vi "ConfirmReceipt.vi"(8 "error in (no error)":errorcluster, 9 "timeout in ms (10000)":i32=10000, 11 "STOMP in":refnum<class "STOMP.lvclass">) -> (0 "error out":errorcluster, 3 "STOMP out":refnum<class "STOMP.lvclass">)   [LabVIEW 2017, in "LabVIEW STOMP.lvlib" / "STOMP.lvclass"]
uses:
  STOMP.lvclass
  STOMP.lvclass/STOMP.ctl
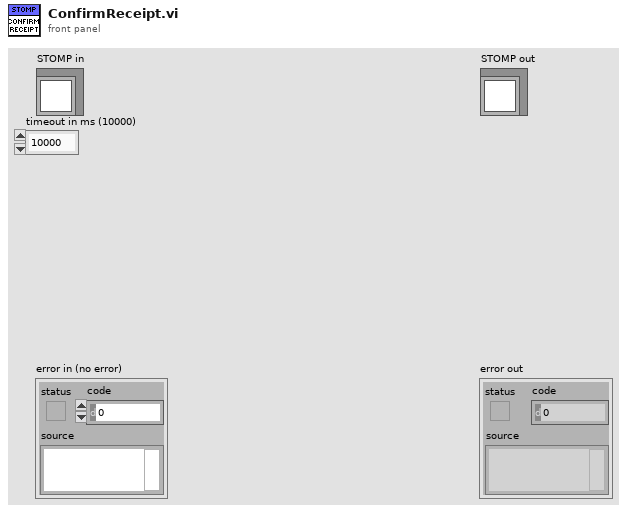
[diagram p1: front panel]
types:
  T1 = typedef "LabVIEW STOMP.lvlib/STOMP.lvclass/Type_ServerFrame.ctl" = cluster{"Type":T2, "Headers":cluster{"Header":string, "Value":string}[], "Body":string}
  T2 = typedef "LabVIEW STOMP.lvlib/STOMP.lvclass/Type_ServerFrameType.ctl" = enum16{"Undefined", "MESSAGE", "CONNECTED", "RECEIPT", "ERROR"}
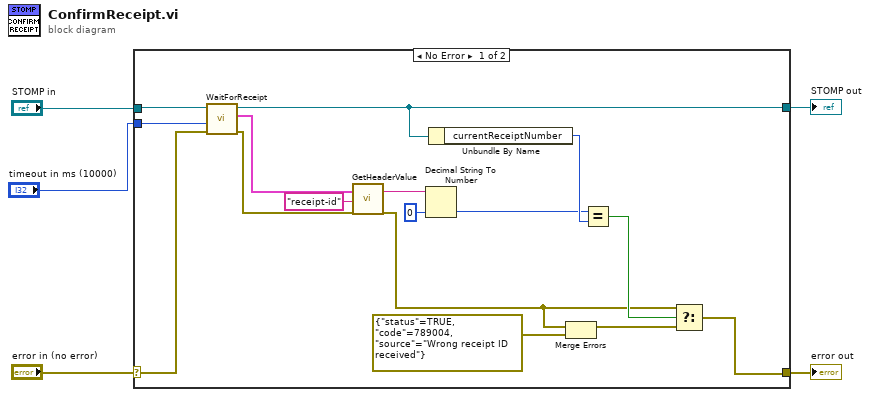
[diagram p0: block diagram]
diagram:
  n1 = case shown="No Error" "error in (no error)" {
    selector: "error in (no error)" -> [w20 w23]
    tunnel: [w6 w23] -> w4
    tunnel: [w14 w22] -> w2
    tunnel: "STOMP in" -> [w21 w22]
    tunnel: "timeout in ms (10000)" -> [w11 _]
    frame No Error {
      n2 = call-dynamic "WaitForReceipt.vi"("error in (no error)"=w20, "timeout in ms (10000)"=w11, "STOMP in"=w21) -> ("error out"=w18:errorcluster, "receipt"=w19:T1, "STOMP out"=w14:refnum<class "STOMP.lvclass">)  [unwired: 6 in]
      n3 = call "GetHeaderValue.vi"("Server Frame"=w19, "Header Name"="receipt-id", "error in"=w18) -> ("Value"=w16:string, "error out"=w9:errorcluster)  [unwired: 15 in]
      n4 = Decimal String To Number(string=w16, default (0L)=u64 0 ("default (0 I32)")) -> (number=w12:u64)  [unwired: 1 in, 1 out]
      n5 = Unbundle By Name(w14) -> ("currentReceiptNumber"=w13:u64)
      n6 = Merge Errors(w9, errorcluster {"status"=TRUE, "code"=789004, "source"="Wrong receipt ID received"} ("error in")) -> (w7:errorcluster)
      n7 = Equal?(x=w12, y=w13) -> (x = y?=w10:bool)
      n8 = Select(t=w9, s=w10, f=w7) -> (s? t:f=w6:errorcluster)
    }
    frame Error {
    }
  }
  "error out" <- w4
  "STOMP out" <- w2
